vi "AlgorithmTimeTester.vi"() -> ()   [LabVIEW 2014]
uses:
  <vilib>/vision/NI_Vision_Development_Module.lvlib
panel:
  in  "Template Path":path
  out "Time Elapsed":dbl
  in  "Image Path":path
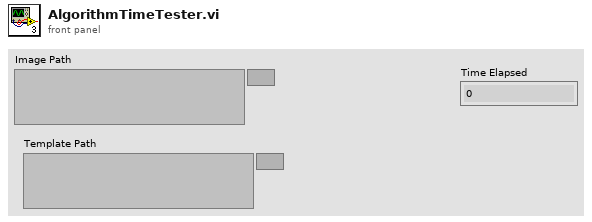
[diagram p1: front panel]
types:
  T1 = typedef "Image Type" = u32
  T2 = typedef "IMAQ Image.ctl" = refnum<image>
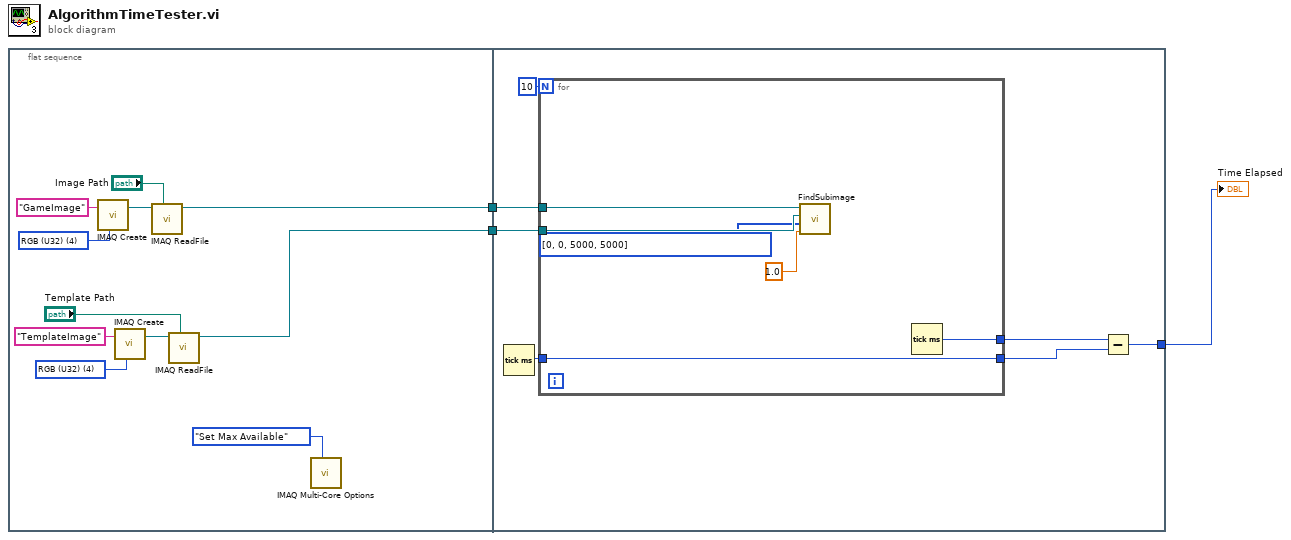
[diagram p0: block diagram]
diagram:
  n1 = flat-sequence {
    tunnel: [w5] -> w2
    tunnel: [w4] -> w1
    tunnel: [w21] -> w3
    tunnel: w2 -> [w16]
    tunnel: w1 -> [w15]
    frame #0 {
      w10 = T1 4 items=["Grayscale (U8)", "Grayscale (I16)", "Grayscale (SGL)", "Complex (CSG)", "RGB (U32)", "HSL (U32)", "RGB (U64)", "Grayscale (U16)"] ("Image Type")
      w14 = T1 4 items=["Grayscale (U8)", "Grayscale (I16)", "Grayscale (SGL)", "Complex (CSG)", "RGB (U32)", "HSL (U32)", "RGB (U64)", "Grayscale (U16)"] ("Image Type")
      n2 = call "IMAQ Create"("Image Name"="GameImage", "Image Type"=w14) -> ("New Image"=w12:T2)  [unwired: 3 in, 1 out]
      n3 = call "IMAQ Create"("Image Name"="TemplateImage", "Image Type"=w10) -> ("New Image"=w8:T2)  [unwired: 3 in, 1 out]
      n4 = call "IMAQ ReadFile"("File Path"="Image Path", "Image"=w12) -> ("Image Out"=w4:T2)  [unwired: 5 in, 4 out]
      n5 = call "IMAQ ReadFile"("File Path"="Template Path", "Image"=w8) -> ("Image Out"=w5:T2)  [unwired: 5 in, 4 out]
      n6 = call "IMAQ Multi-Core Options"("Get/Set Number of Cores (Get)"=enum32{"Get", "Set", "Set Max Available"}."Set Max Available") -> ()  [unwired: 9 in, 2 out]
    }
    frame #1 {
      n7 = Tick Count (ms)() -> (millisecond timer value=w20:u32)
      n8 = for {
        N: 10 -> [_]
        tunnel: [w27] -> w18
        tunnel: w20 -> [w27]
        tunnel: [w26] -> w19
        tunnel: w16 -> [w24]
        tunnel: w15 -> [w25]
        n9 = call "FindSubimage.vi"("Scale factor (1)"=1.0, "ROI (left top right bottom)"=u32[] [0, 0, 5000, 5000], "RGB Template"=w24, "RGB Image"=w25) -> ()  [unwired: 7 in, 1 out]
        n10 = Tick Count (ms)() -> (millisecond timer value=w26:u32)
      }
      n11 = Subtract(x=w19, y=w18) -> (x-y=w21:u32)
    }
  }
  "Time Elapsed" <- w3
